vi "Read String.vi"(8 "error in (no error)":errorcluster, 9 "Timeout (ms)":i32, 11 "CIFTag in":refnum<class "CIF_CIPC_Chn_String.lvclass">) -> (0 "error out":errorcluster, 1 "timed out?":bool, 2 "Data":string, 3 "CIFTag out":refnum<class "CIF_CIPC_Chn_String.lvclass">)   [LabVIEW 2021, in "CIF_CIPC_Chn_String.lvclass"]
uses:
  CIF_CIPC_Chn_String.lvclass
  D:/dev/Packages/CIF_Channels_Core/src/CIFChannels/CIFChannels.lvclass
  D:/dev/Packages/CIF_Channels_Core/src/CIPC_Channels/CIF_CIPC_Chan/CIF_CIPC_Chn.lvclass
  CIFChannels/CIFChannels.lvclass/CIFChannels.ctl
  CIF_CIPC_Chn_String.lvclass/CIF_CIPC_Chn_String.ctl
  CIF_CIPC_Chan/CIF_CIPC_Chn.lvclass/CIF_CIPC_Chn.ctl
  CIF_CIPC_Chan/Accessors/Read CIPC Channel.vi
  CIF_CIPC_Chan/SubVIs/Check Disconnect.vi
  Read String Direct.vi/ed3b2614-2534-48bf-9d55-8103b1731be4.vi
  Read String Direct.vi/9835d51f-0a03-4fca-8b65-57ff329e3dc0.vi
  CIF_CIPC_Chan/Accessors/Read Buffer Configuration.vi
  CIF_CIPC_Chan/Accessors/Read Data Type.vi
  CIFChannels/Accessors/Read Channel State.vi
  CIFChannels/Accessors/Read Direction.vi
  CIFChannels/Accessors/Read Tag Forced.vi
  CIFChannels/Accessors/Write Channel State.vi
  CIFChannels/Accessors/Read Tag Disconnect Behavior.vi
  <vilib>/CIF Foundation/CIF CIPC/SubVIs/Wait For N Elements Available.vi
  <vilib>/CIF Foundation/CIF CIPC/SubVIs/Get Element Read Position.vi
  <vilib>/CIF Foundation/CIF CIPC/SubVIs/Check Error.vi
  <vilib>/CIF Foundation/CIF CIPC/SubVIs/Get dll Path.vi
  <vilib>/CIF Foundation/CIF CIPC/SubVIs/Set Element Read Position.vi
  CIF_CIPC_Chan/CIF_CIPC_Chn.lvclass
  <vilib>/Utility/error.llb/Trim Whitespace.vi
  <vilib>/Utility/error.llb/Error Cluster From Error Code.vi
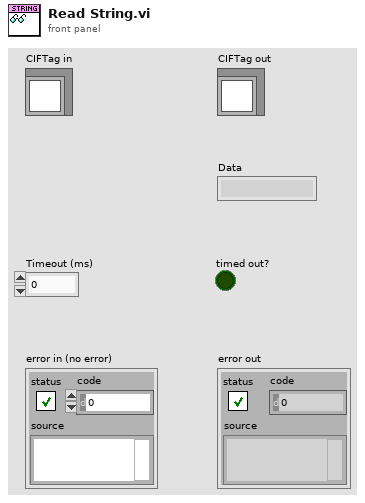
[diagram p1: front panel]
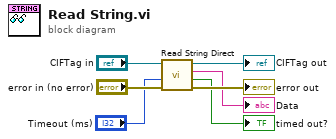
[diagram p0: block diagram]
diagram:
  n1 = call "Read String Direct.vi"("error in (no error)"="error in (no error)", "Timeout (ms)"="Timeout (ms)", "CIFTag in"="CIFTag in") -> ("error out"=→"error out":errorcluster, "timed out?"=→"timed out?":bool, "Data"=→"Data":string, "CIFTag out"=→"CIFTag out":refnum<class "CIF_CIPC_Chn_String.lvclass">)  [unwired: 5 in]
